vi "Create and Save Signal.vi"   [LabVIEW 2015]
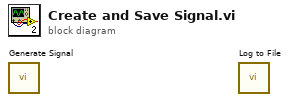
[diagram p0: block diagram]
diagram:
  n1 = call "Generate Signal.vi"() -> ()  [unwired: 1 in]
  n2 = call "Log to File.vi"() -> ()  [unwired: 1 in]
